vi "FTW-CodeGen-GetHelp.vi"(0 "State In":T4, 5 "XRef":refnum<vi>, 7 "Point":cluster{"Horizontal":i32, "Vertical":i32}) -> (4 "Standard Help Info":T3, 6 "Detailed Help Info":T2, 8 "Subitem Help Info":T1, 10 "Use Detailed Help?":bool, 15 "Use Subitem Help?":bool)   [LabVIEW 2015, in "FTW-Dataflow-Burrow.xnode"]
uses:
  FTW-Dataflow-Burrow.xnode
  FTW-CodeGen-State.ctl
panel:
  # "Inputs"
  # "Outputs"
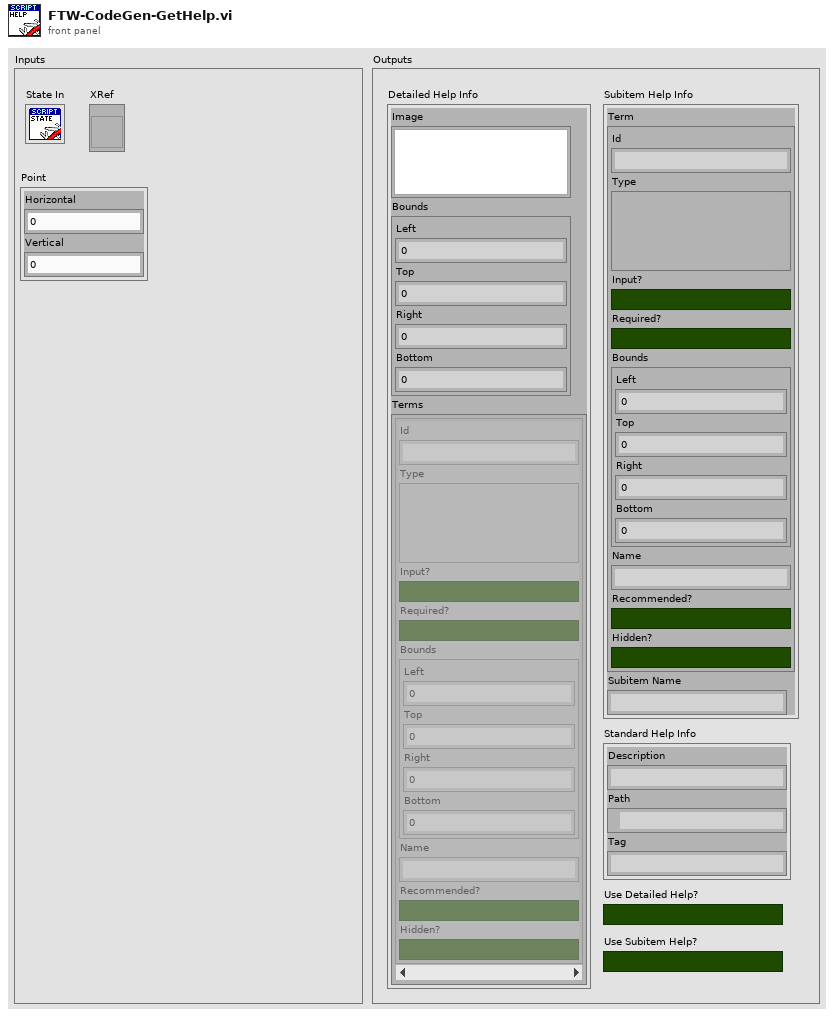
[diagram p1: front panel]
types:
  T1 = cluster{"Term":cluster{"Id":string, "Type":variant, "Input?":bool, "Required?":bool, "Bounds":cluster{"Left":i32, "Top":i32, "Right":i32, "Bottom":i32}, "Name":string, "Recommended?":bool, "Hidden?":bool}, "Subitem Name":string}
  T2 = cluster{"Image":picture, "Bounds":cluster{"Left":i32, "Top":i32, "Right":i32, "Bottom":i32}, "Terms":cluster{"Id":string, "Type":variant, "Input?":bool, "Required?":bool, "Bounds":cluster{"Left":i32, "Top":i32, "Right":i32, "Bottom":i32}, "Name":string, "Recommended?":bool, "Hidden?":bool}[]}
  T3 = cluster{"Description":string, "Path":path, "Tag":string}
  T4 = typedef "FTW-Dataflow-Burrow.xnode/FTW-CodeGen-State.ctl" = cluster{"InputTerminals":cluster{"Wired?":bool, "ID":string, "DataName":string, "DataColor":u32, "Type":variant}[], "EnableTiming?":bool}
  T5 = cluster{"Id":string, "Type":variant, "Input?":bool, "Required?":bool, "Bounds":cluster{"Left":i32, "Top":i32, "Right":i32, "Bottom":i32}, "Name":string, "Recommended?":bool, "Hidden?":bool}
  T6 = cluster{"Name":string, "Id":string, "Type":variant, "Bounds":cluster{"Left":i32, "Top":i32, "Right":i32, "Bottom":i32}, "Input?":bool, "Required?":bool, "Recommended?":bool, "Adaptive?":bool, "Hidden?":bool, "Direction":enum32{"Auto", "Up", "Down", "Left", "Right", "Center"}, "Break Wire?":bool, "English Name":string}[]
  T7 = cluster{"Left":i32, "Top":i32, "Right":i32, "Bottom":i32}
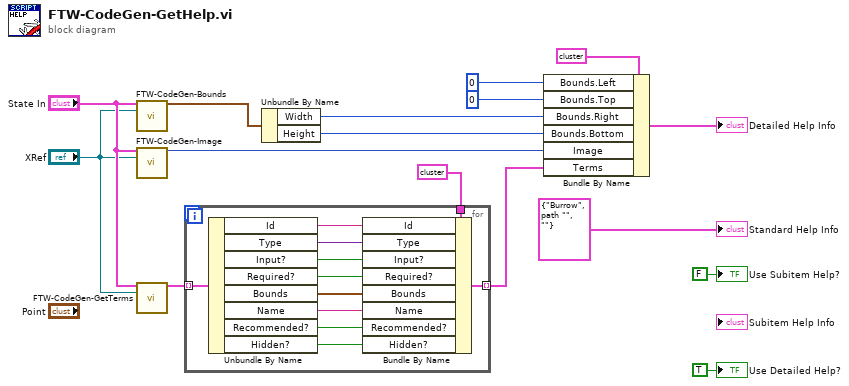
[diagram p0: block diagram]
diagram:
  n1 = call "FTW-CodeGen-Bounds.vi"("State In"="State In", "XRef"="XRef") -> ("Bounds"=w8:cluster{"Width":i32, "Height":i32})  [unwired: 13 in]
  n2 = call "FTW-CodeGen-Image.vi"("State In"="State In", "XRef"="XRef") -> ("Image"=w13:picture)  [unwired: 13 in]
  n3 = call "FTW-CodeGen-GetTerms.vi"("State In"="State In", "XRef"="XRef") -> ("Terms"=w10:T6)  [unwired: 13 in]
  n4 = for {
    tunnel: [w26] -> w12 mode=indexing
    tunnel: T5 {"Id"="", "Type"=variant, "Input?"=FALSE, "Required?"=FALSE, "Bounds"={"Left"=0, "Top"=0, "Right"=0, "Bottom"=0}, "Name"="", "Recommended?"=FALSE, "Hidden?"=FALSE} ("Term") -> [w27]
    tunnel: w10 -> [w25] mode=indexing
    n5 = Unbundle By Name(w25) -> ("Id"=w24:string, "Type"=w23:variant, "Input?"=w22:bool, "Required?"=w21:bool, "Bounds"=w20:T7, "Name"=w19:string, "Recommended?"=w18:bool, "Hidden?"=w17:bool)
    n6 = Bundle By Name(cluster=w27, "Id"=w24, "Type"=w23, "Input?"=w22, "Required?"=w21, "Bounds"=w20, "Name"=w19, "Recommended?"=w18, "Hidden?"=w17) -> (w26:T5)
  }
  n7 = Unbundle By Name(w8) -> ("Width"=w2:i32, "Height"=w3:i32)
  n8 = Bundle By Name(cluster=T2 {"Image"=bytes[0], "Bounds"={"Left"=0, "Top"=0, "Right"=0, "Bottom"=0}, "Terms"=[]} ("Detailed Help Info"), "Bounds.Left"=0, "Bounds.Top"=0, "Bounds.Right"=w2, "Bounds.Bottom"=w3, "Image"=w13, "Terms"=w12) -> (→"Detailed Help Info":T2)
  "Standard Help Info" <- T3 {"Description"="Burrow", "Path"=path "", "Tag"=""} ("Standard Help Info")
  "Use Detailed Help?" <- TRUE ("Use Detailed Help?")
  "Use Subitem Help?" <- FALSE ("Use Subitem Help?")
